vi "Split Array Even-Odd.vi"(11 "Input Array":i32[][](array[numeric])) -> (2 "Out Array 2":i32[][](array[numeric]), 3 "Out Array 1":i32[][](array[numeric]))   [LabVIEW 2012]
panel:
  # "From Input Array, puts all even rows into Out Array 1\nand all odd rows into Out Array 2"
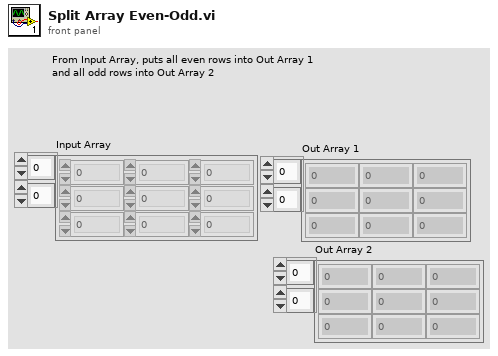
[diagram p1: front panel]
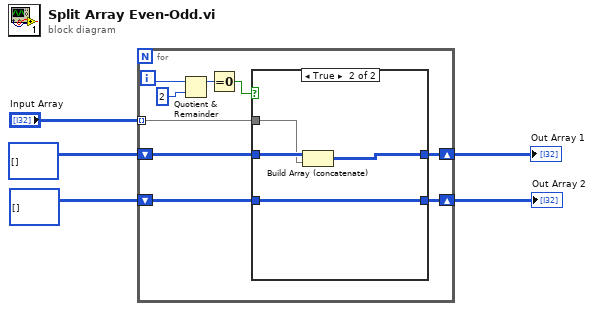
[diagram p0: block diagram]
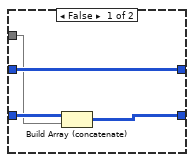
[diagram p2: hidden frame]
diagram:
  n1 = for {
    tunnel: "Input Array" -> [w10] mode=indexing
    shift-right: [w9] -> w2
    shift-left: i32[][] [] ("Input Array 2") -> [w12]
    shift-right: [w8] -> w1
    shift-left: i32[][] [] ("Input Array 2") -> [w11]
    i -> [w6]
    n2 = Quotient & Remainder(x=w6, y=2) -> (x-y*floor(x/y)=w7:i32)  [unwired: 1 out]
    n3 = Equal To 0?(x=w7) -> (x = 0?=w13:bool)
    n4 = case shown="True" w13 {
      tunnel: w12 -> [w17 w22]
      tunnel: w11 -> [w16 w19]
      tunnel: w10 -> [w15 w21]
      tunnel: [w17 w20] -> w9
      tunnel: [w18 w19] -> w8
      frame False {
        n5 = Build Array (concatenate)(w16, w15) -> (w18:i32[][])
      }
      frame True {
        n6 = Build Array (concatenate)(w22, w21) -> (w20:i32[][])
      }
    }
  }
  "Out Array 1" <- w2
  "Out Array 2" <- w1
